vi "data_out.vi"(8 "error in (no error)":errorcluster, 11 "Counter in":refnum<class "Counter.lvclass">) -> (0 "error out":errorcluster, 2 "counter data string":string, 3 "Counter out":refnum<class "Counter.lvclass">)   [LabVIEW 2014, in "Counter.lvclass"]
uses:
  Counter.lvclass
  Counter.lvclass/Counter.ctl
  Globals.vi
  TCP_IP/TCP_IP.lvclass
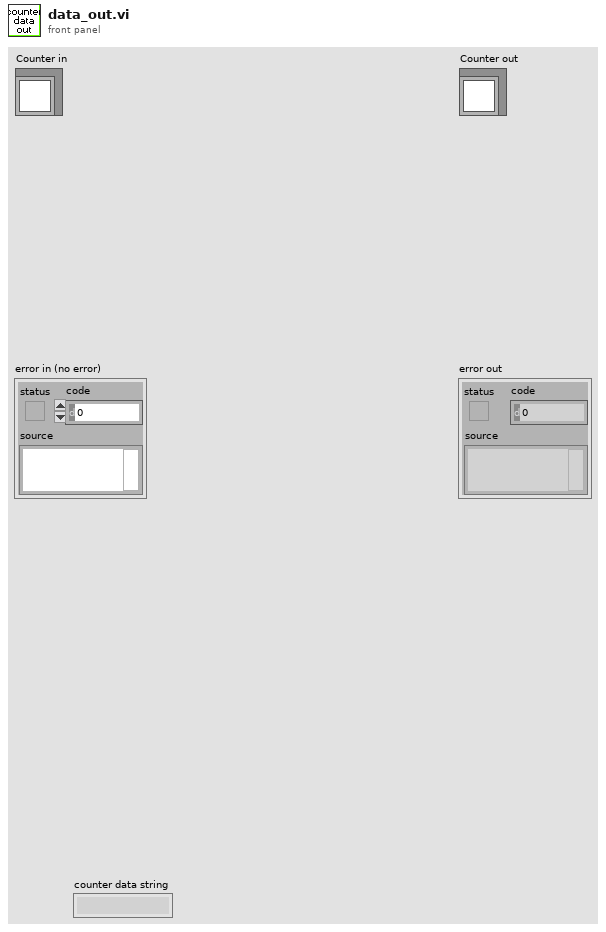
[diagram p1: front panel]
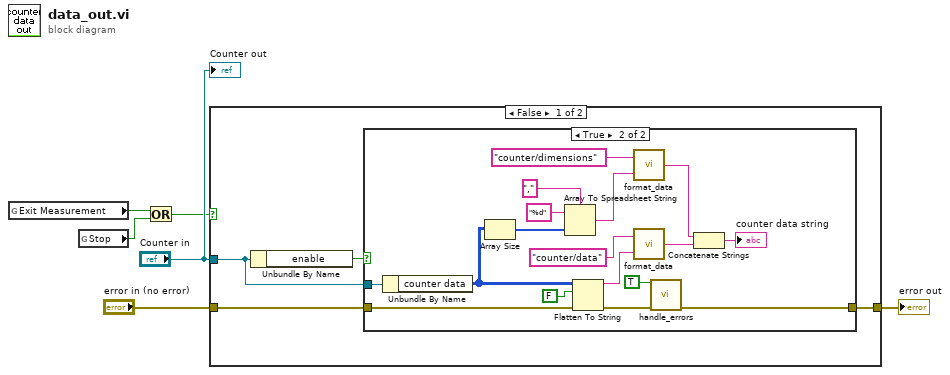
[diagram p0: block diagram]
diagram:
  n1 = global read "Globals.vi" "Exit Measurement"() -> (w5:bool)
  n2 = global read "Globals.vi" "Stop"() -> (w4:bool)
  n3 = Or(x=w5, y=w4) -> (x .or. y?=w3:bool)
  n4 = case shown="False" w3 {
    tunnel: "Counter in" -> [w9 _]
    tunnel: "error in (no error)" -> [w8 w29]
    tunnel: [w7 w29] -> w1
    frame False {
      n5 = Unbundle By Name(w9) -> ("enable"=w10:bool)
      n6 = case shown="True" w10 {
        tunnel: w9 -> [_ w19]
        tunnel: w8 -> [w11 w15]
        tunnel: [w11 w13] -> w7
        frame False {
        }
        frame True {
          n7 = Unbundle By Name(w19) -> ("counter data"=w18:u32[][])
          n8 = Array Size(array=w18) -> (size(s)=w26:i32[])
          n9 = Array To Spreadsheet String(delimiter (Tab)=",", array=w26, 3:"%d" ("format string")) -> (spreadsheet string=w24:string)
          n10 = Flatten To String(anything=w18, prepend array or string size? (T)=FALSE, error in (no error)=w15) -> (data string=w16:string, error out=w14:errorcluster)  [unwired: 1 in, 1 out]
          n11 = call "format_data.vi"("data"=w24, "name"="counter/dimensions") -> ("concatenated string"=w22:string)
          n12 = call "format_data.vi"("data"=w16, "name"="counter/data") -> ("concatenated string"=w21:string)
          n13 = call "handle_errors.vi"("Exit Operation"=TRUE, "error in (no error)"=w14) -> ("error out"=w13:errorcluster)  [unwired: 13 in]
          n14 = Concatenate Strings(w22, w21) -> (→"counter data string":string)
        }
      }
    }
    frame True {
    }
  }
  "error out" <- w1
  "Counter out" <- "Counter in"
